vi "SaveMouseROI.vi"(7 "BlockFolderPath":path, 9 "File Path for Mouse Mask":path, 10 "sessionID":string, 11 "MouseRoi Refnum in":T1) -> ()   [LabVIEW 2013]
uses:
  <vilib>/vision/Image Controls.llb/IMAQ Image.ctl
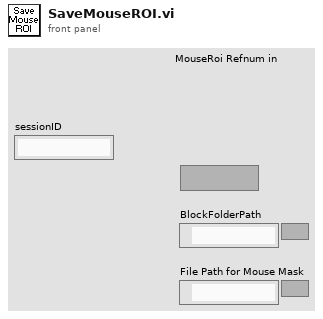
[diagram p1: front panel]
types:
  T1 = typedef "IMAQ Image.ctl" = refnum<image>
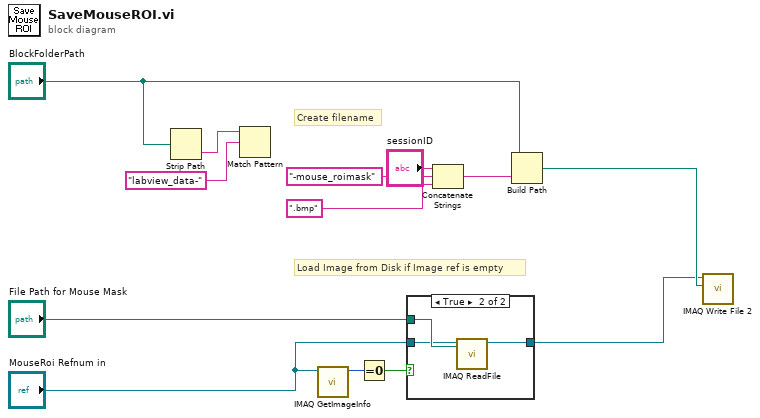
[diagram p0: block diagram]
diagram:
  # "Load Image from Disk if Image ref is empty"
  # "Create filename"
  n1 = Strip Path(path="BlockFolderPath") -> (name=w3:string)  [unwired: 1 out]
  n2 = Match Pattern(string=w3, regular expression="labview_data-") -> ()  [unwired: 1 in, 4 out]
  n3 = call "IMAQ GetImageInfo"("Image"="MouseRoi Refnum in") -> ("X Resolution"=w7:i32)  [unwired: 3 in, 7 out]
  n4 = Equal To 0?(x=w7) -> (x = 0?=w6:bool)
  n5 = case shown="True" w6 {
    tunnel: "File Path for Mouse Mask" -> [_ w17]
    tunnel: "MouseRoi Refnum in" -> [w14 w16]
    tunnel: [w14 w15] -> w10
    frame False {
    }
    frame True {
      n6 = call "IMAQ ReadFile"("File Path"=w17, "Image"=w16) -> ("Image Out"=w15:T1)  [unwired: 5 in, 4 out]
    }
  }
  n7 = Concatenate Strings("sessionID", "-mouse_roimask" ("string"), ".bmp" ("string")) -> (w12:string)
  n8 = Build Path(base path="BlockFolderPath", name or relative path=w12) -> (appended path=w13:path)
  n9 = call-poly "IMAQ Write File 2"("File Path"=w13, "Image"=w10) -> ()  [unwired: 8 in, 2 out]
